vi "Pointer_Determine Intersection.vi"(8 "Error":errorcluster, 9 "WAvIndex Pointer  Two":refnum<class "WavIndex_Pointer.lvclass">, 11 "WAvIndex Pointer One":refnum<class "WavIndex_Pointer.lvclass">) -> (0 "Error Out":errorcluster, 3 "Intersection Type Out":T1)   [LabVIEW 2020, in "WavBuf.lvclass"]
doc: "Determines the type of time intersection"
uses:
  WavBuf/WavBuf.lvclass
  Pointer/WavIndex_Pointer/WavIndex_Pointer.lvclass
  TypeDefs_Utility/ENUM_Intersection type.ctl
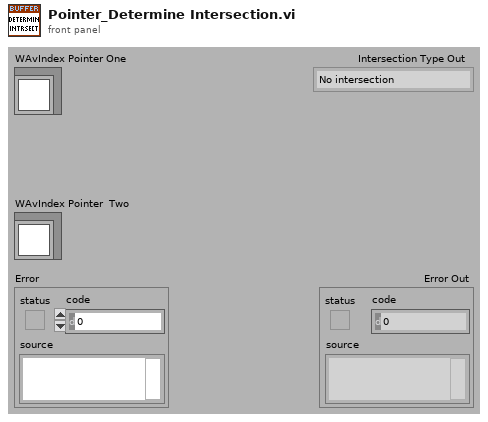
[diagram p1: front panel]
types:
  T1 = typedef "ENUM_Intersection type.ctl" = enum16{"No intersection", "Interleave 1 later than 2", "Interleave 2 later than 1", "Engulf 1 around 2", "Engulf 2 around 1"}
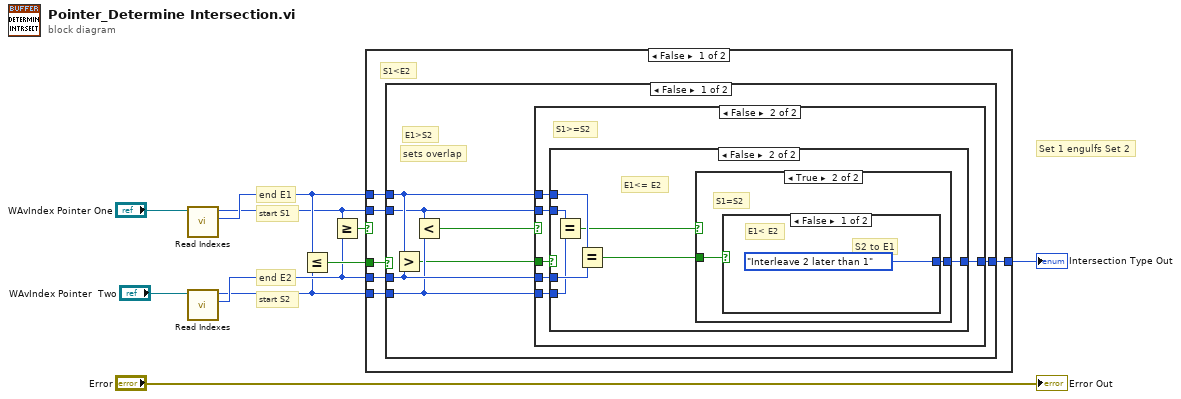
[diagram p0: block diagram]
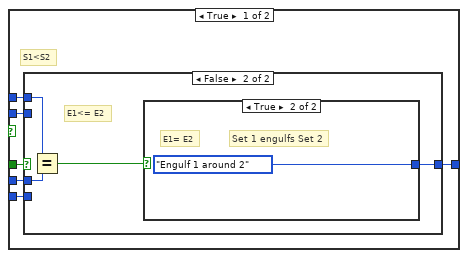
[diagram p2: hidden frame]
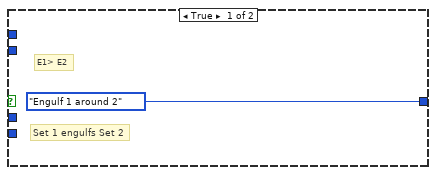
[diagram p3: hidden frame]
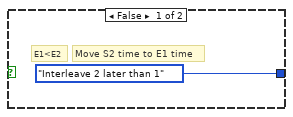
[diagram p4: hidden frame]
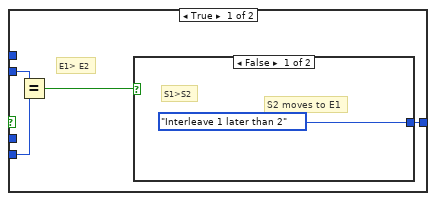
[diagram p5: hidden frame]
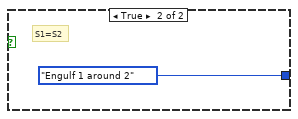
[diagram p6: hidden frame]
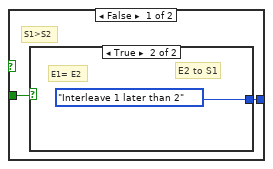
[diagram p7: hidden frame]
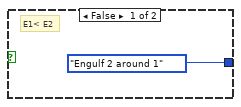
[diagram p8: hidden frame]
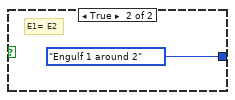
[diagram p9: hidden frame]
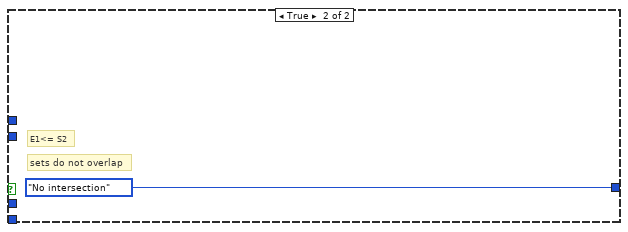
[diagram p10: hidden frame]
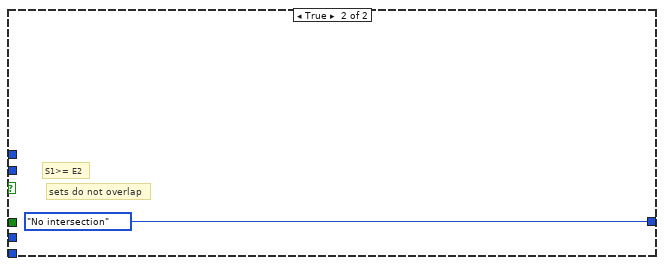
[diagram p11: hidden frame]
diagram:
  # "Set 1 engulfs Set 2"
  # "end E2"
  # "start S2"
  # "start S1"
  # "end E1"
  n1 = call "Read Indexes.vi"("(WavIndex_Pointer)"="WAvIndex Pointer One") -> ("End Out"=w5:i32, "Start Out"=w4:i32)  [unwired: 9 in]
  n2 = call "Read Indexes.vi"("(WavIndex_Pointer)"="WAvIndex Pointer  Two") -> ("End Out"=w2:i32, "Start Out"=w1:i32)  [unwired: 9 in]
  n3 = Less Or Equal?(x=w5, y=w1) -> (x <= y?=w8:bool)
  n4 = Greater Or Equal?(x=w4, y=w2) -> (x >= y?=w7:bool)
  n5 = case shown="False" w7 {
    tunnel: w8 -> [w16 _]
    tunnel: w1 -> [w15 _]
    tunnel: w2 -> [w14 _]
    tunnel: w4 -> [w13 _]
    tunnel: w5 -> [w12 _]
    tunnel: [w11 ENUM_Intersection_type."No intersection" ("Intersection Type")] -> w9
    frame False {
      # "S1<E2"
      n6 = case shown="False" w16 {
        tunnel: w15 -> [w20 _]
        tunnel: w14 -> [w23 _]
        tunnel: w13 -> [w21 _]
        tunnel: w12 -> [w22 _]
        tunnel: [w19 ENUM_Intersection_type."No intersection" ("Intersection Type")] -> w11
        frame False {
          # "sets overlap"
          # "E1>S2"
          n7 = Greater?(x=w22, y=w23) -> (0:w18:bool)
          n8 = Less?(x=w21, y=w20) -> (x < y?=w17:bool)
          n9 = case shown="False" w17 {
            tunnel: w18 -> [w29 w42]
            tunnel: w23 -> [w28 w39]
            tunnel: w22 -> [w27 w38]
            tunnel: w21 -> [w26 w41]
            tunnel: w20 -> [w25 w40]
            tunnel: [w24 w37] -> w19
            frame True {
              # "S1<S2"
              n10 = case shown="False" w29 {
                tunnel: w28 -> [_ w33]
                tunnel: w27 -> [_ w34]
                tunnel: w26 -> [_ _]
                tunnel: w25 -> [_ _]
                tunnel: [ENUM_Intersection_type."Engulf 1 around 2" ("Intersection Type") w32] -> w24
                frame True {
                  # "Set 1 engulfs Set 2"
                  # "E1> E2"
                }
                frame False {
                  # "E1<= E2"
                  n11 = Equal?(x=w34, y=w33) -> (x = y?=w31:bool)
                  n12 = case shown="True" w31 {
                    tunnel: [ENUM_Intersection_type."Interleave 2 later than 1" ("Intersection Type") ENUM_Intersection_type."Engulf 1 around 2" ("Intersection Type")] -> w32
                    frame False {
                      # "Move S2 time to E1 time"
                      # "E1<E2"
                    }
                    frame True {
                      # "Set 1 engulfs Set 2"
                      # "E1= E2"
                    }
                  }
                }
              }
            }
            frame False {
              # "S1>=S2"
              n13 = case shown="False" w42 {
                tunnel: w41 -> [w46 w52]
                tunnel: w40 -> [w45 w54]
                tunnel: w39 -> [_ w55]
                tunnel: w38 -> [_ w53]
                tunnel: [w44 w51] -> w37
                frame True {
                  # "E1> E2"
                  n14 = Equal?(x=w46, y=w45) -> (x = y?=w43:bool)
                  n15 = case shown="False" w43 {
                    tunnel: [ENUM_Intersection_type."Interleave 1 later than 2" ("Intersection Type Out") ENUM_Intersection_type."Engulf 1 around 2" ("Intersection Type Out")] -> w44
                    frame False {
                      # "S2 moves to E1"
                      # "S1>S2"
                    }
                    frame True {
                      # "S1=S2"
                    }
                  }
                }
                frame False {
                  # "E1<= E2"
                  n16 = Equal?(x=w52, y=w54) -> (x = y?=w50:bool)
                  n17 = Equal?(x=w53, y=w55) -> (x = y?=w49:bool)
                  n18 = case shown="True" w50 {
                    tunnel: w49 -> [w57 w61]
                    tunnel: [w56 w60] -> w51
                    frame False {
                      # "S1>S2"
                      n19 = case shown="True" w57 {
                        tunnel: [ENUM_Intersection_type."Engulf 2 around 1" ("Intersection Type Out") ENUM_Intersection_type."Interleave 1 later than 2" ("Intersection Type Out")] -> w56
                        frame False {
                          # "E1< E2"
                        }
                        frame True {
                          # "E2 to S1"
                          # "E1= E2"
                        }
                      }
                    }
                    frame True {
                      # "S1=S2"
                      n20 = case shown="False" w61 {
                        tunnel: [ENUM_Intersection_type."Interleave 2 later than 1" ("Intersection Type Out") ENUM_Intersection_type."Engulf 1 around 2" ("Intersection Type Out")] -> w60
                        frame False {
                          # "S2 to E1"
                          # "E1< E2"
                        }
                        frame True {
                          # "E1= E2"
                        }
                      }
                    }
                  }
                }
              }
            }
          }
        }
        frame True {
          # "sets do not overlap"
          # "E1<= S2"
        }
      }
    }
    frame True {
      # "sets do not overlap"
      # "S1>= E2"
    }
  }
  "Intersection Type Out" <- w9
  "Error Out" <- "Error"
